vi "Write VI Refnum.vi"(8 "error in (no error)":errorcluster, 10 "VI Refnum":refnum<vi>, 11 "Mensajes in":refnum<class "Mensajes.lvclass">) -> (0 "error out":errorcluster, 3 "Mensajes out":refnum<class "Mensajes.lvclass">)   [LabVIEW 2019, in "Mensajes.lvlib" / "Mensajes.lvclass"]
uses:
  Mensajes.lvclass
  Mensajes.lvclass/Mensajes.ctl
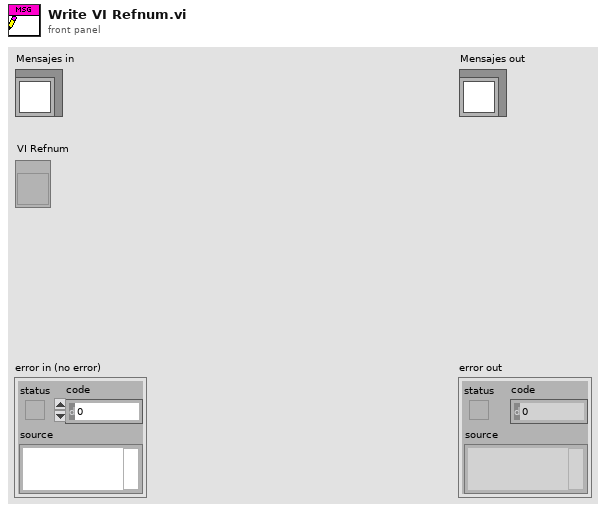
[diagram p1: front panel]
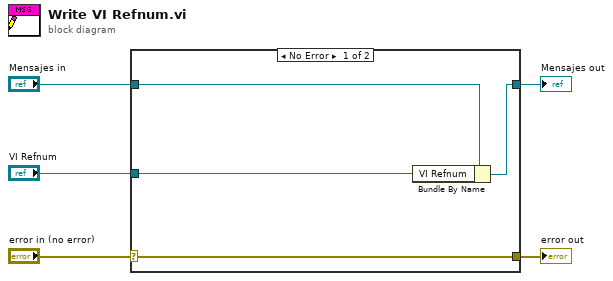
[diagram p0: block diagram]
diagram:
  n1 = case shown="No Error" "error in (no error)" {
    selector: "error in (no error)" -> [w9 w10]
    tunnel: [w9 w10] -> w4
    tunnel: [w7 w11] -> w2
    tunnel: "Mensajes in" -> [w8 w11]
    tunnel: "VI Refnum" -> [w6 _]
    frame No Error {
      n2 = Bundle By Name(cluster=w8, "VI Refnum"=w6) -> (w7:refnum<class "Mensajes.lvclass">)
    }
    frame Error {
    }
  }
  "error out" <- w4
  "Mensajes out" <- w2
